vi "PH_SRDG645.evt Call Close.vi"(0 "i ref in":refnum<vi>, 1 "Generator Instance":string="N/A", 5 "error IO":errorcluster) -> (14 "i ref out":refnum<vi>, 19 "error out":errorcluster)   [LabVIEW 2014, in "PH_SRDG645.lvlib"]
doc: "This VI sends a simple event call."
uses:
  PH_SRDG645.lvlib
  CSCore/BaseProcess/BaseProcess.lvlib
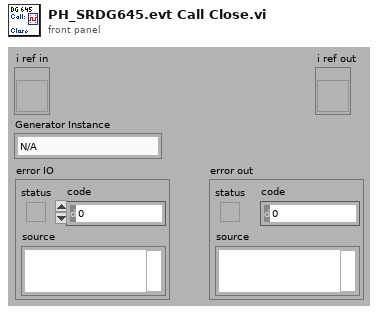
[diagram p1: front panel]
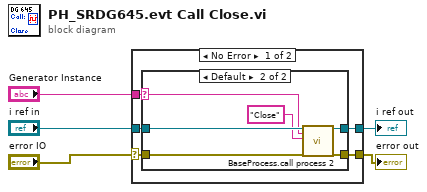
[diagram p0: block diagram]
diagram:
  n1 = case shown="No Error" "error IO" {
    selector: "error IO" -> [w10 w19]
    tunnel: "Generator Instance" -> [w6 _]
    tunnel: [w9 w19] -> w5
    tunnel: [w7 w20] -> w4
    tunnel: "i ref in" -> [w8 w20]
    frame No Error {
      n2 = case shown="Default" w6 {
        selector: w6 -> [_ w13]
        tunnel: w10 -> [w11 w18]
        tunnel: [w11 w17] -> w9
        tunnel: w8 -> [w12 w16]
        tunnel: [w12 w15] -> w7
        frame "", "N/A" {
        }
        frame Default {
          n3 = call "BaseProcess.call process 2.vi"("i ref in"=w16, "Object"=w13, "Selector"="Close", "error in (no error)"=w18) -> ("i ref out"=w15:refnum<vi>, "error out"=w17:errorcluster)  [unwired: 14 in]
        }
      }
    }
    frame Error {
    }
  }
  "error out" <- w5
  "i ref out" <- w4
